vi "Write Image.vi"(8 "error in (no error)":errorcluster, 10 "Image":picture, 11 "_Popup in":refnum<class "Popup.lvclass">) -> (0 "error out":errorcluster, 3 "_Popup out":refnum<class "Popup.lvclass">)   [LabVIEW 2021, in "Pop-Up.lvlib" / "Popup.lvclass"]
doc: "This Data Member Access VI will write the Image to the object.\n\nInputs: +\n-Image [2D Picture] - the image to write to the display pop up\n\n<b>Code Developed By:</b> +\nDaniel Coons +\nhttps://github.com/danielcoons/tsc-pop-up"
uses:
  Popup.lvclass
  Popup.lvclass/Popup.ctl
panel:
  # "This VI puts the Image value (PNG Graphic) into the Popup Object"
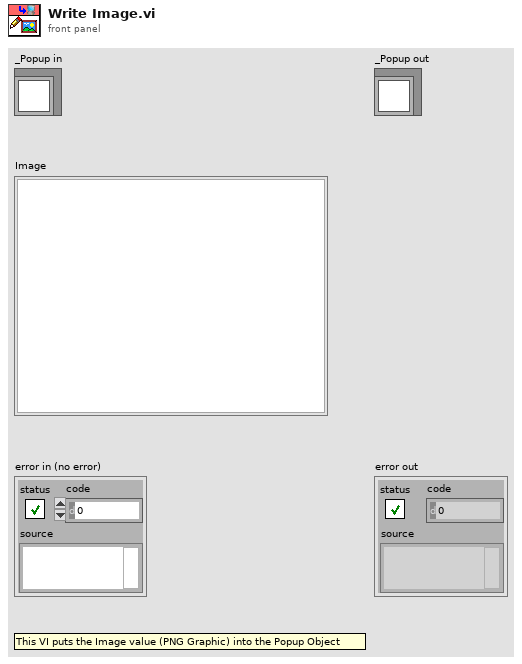
[diagram p1: front panel]
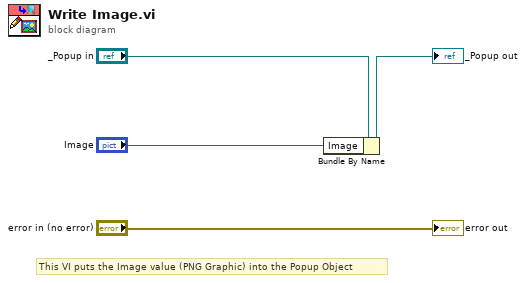
[diagram p0: block diagram]
diagram:
  # "This VI puts the Image value (PNG Graphic) into the Popup Object"
  n1 = Bundle By Name(cluster="_Popup in", "Image"="Image") -> (→"_Popup out":refnum<class "Popup.lvclass">)
  "error out" <- "error in (no error)"
